vi "Config.vi"(8 "error in (no error)":errorcluster, 10 "Setting":variant, 11 "Lambda Gen LAN in":refnum<class "Lambda Gen LAN.lvclass">) -> (0 "error out":errorcluster, 3 "Lambda Gen LAN out":refnum<class "Lambda Gen LAN.lvclass">)   [LabVIEW 2025, in "Power Supply.lvlib" / "Lambda Gen LAN.lvclass"]
uses:
  Lambda Gen LAN.lvclass
  C:/Users/Public/Documents/Sandia National Labs/TSS Plugin/CEF.lvlibp/Node/CEF_Node.lvclass
  C:/Users/Public/Documents/Sandia National Labs/TSS Plugin/Abstract Engine.lvlibp/Abstract Instrument/Abstract Instrument.lvclass
  PS Channel/Power Supply Channel.lvclass
  Users/Public/Documents/Sandia National Labs/TSS Plugin/Abstract Engine.lvlibp/Abstract Instrument/Channel.ctl
  Lambda Gen LAN.lvclass/Lambda Gen LAN.ctl
  PS Channel configuration/Power Supply Channel configuration.lvclass
  C:/Users/Public/Documents/Sandia National Labs/TSS Plugin/Abstract Engine.lvlibp/Channel configuration/Channel configuration.lvclass
  PS Channel configuration/Power Supply Channel configuration.lvclass/Power Supply Channel configuration.ctl
  PS Channel configuration/Read PS Channel.vi
  Users/Public/Documents/Sandia National Labs/TSS Plugin/CEF.lvlibp/Node/ReadChildren.vi
  Users/Public/Documents/Sandia National Labs/TSS Plugin/Abstract Engine.lvlibp/Channel configuration/Read Channel Setting.vi
  Users/Public/Documents/Sandia National Labs/TSS Plugin/CEF.lvlibp/Node/CEF_Node.lvclass
  Users/Public/Documents/Sandia National Labs/TSS Plugin/CEF.lvlibp/serializable configuration/CEF_serializable configuration.lvclass
  <instrlib>/TDK-Lambda GEN LAN Series/TDK-Lambda GEN LAN Series.lvlib
  Users/Public/Documents/Sandia National Labs/TSS Plugin/Abstract Engine.lvlibp/Abstract Instrument/Abstract Instrument.lvclass
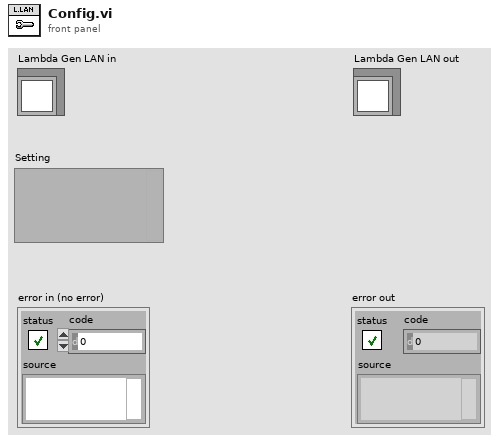
[diagram p1: front panel]
types:
  T1 = typedef "Abstract Engine.lvlibp/Abstract Instrument.lvclass/Channel.ctl" = cluster{"Alias":string, "DataType":enum16{"Anaolg Input", "Waveform"}, "Unit":enum16{"---", "V", "A", "Ohm", "Hz", "uF", "degC", "deg"}, "Upper limit":dbl, "Lower limit":dbl, "Measurement":variant}
  T2 = typedef "Abstract Engine.lvlibp/Channel configuration.lvclass/Default Channel.ctl" = cluster{"Address":string, "SW Alias":string, "Enabled":bool, "Type":string, "Description":string}
  T3 = typedef "Power Supply.lvlib/Power Supply Channel configuration.lvclass/PS Channel Setting.ctl" = cluster{"Driver":string, "Pin":string, "Test Voltage":string, "Voltage Low":dbl, "Voltage Norminal":dbl, "Voltage High":dbl, "PreTest Voltage":dbl, "PreTest Current":dbl, "Current Limit":dbl}
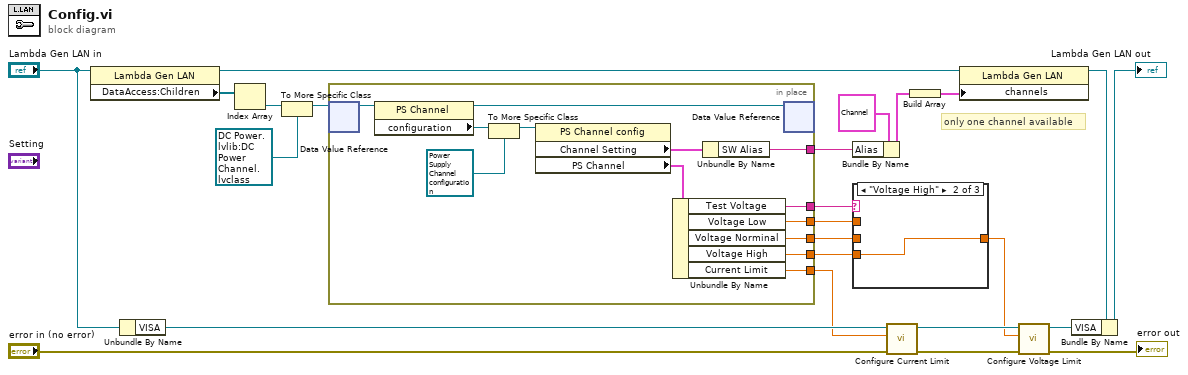
[diagram p0: block diagram]
diagram:
  # "only one channel available"
  n1 = property class="Lambda Gen LAN"(reference="Lambda Gen LAN in") -> (reference out=w18:refnum<class "Lambda Gen LAN.lvclass">, "DataAccess:Children"=w17:refnum<data-value>[])  [unwired: 1 in, 1 out]
  n2 = Unbundle By Name("Lambda Gen LAN in") -> ("VISA"=w23:refnum<visa-resource-name>)
  n3 = Index Array(array=w17) -> (element=w16:refnum<data-value>)  [unwired: 1 in]
  n4 = To More Specific Class(target class=refnum<data-value> refnum ("data value reference"), reference=w16) -> (specific class reference=w15:refnum<data-value>)  [unwired: 1 in, 1 out]
  n5 = in-place {
    in-place-border: [w29] -> w10
    in-place-border: [w30] -> w8
    in-place-border: [w28] -> w7
    in-place-border: [w27] -> w6
    in-place-border: [w26] -> w4
    in-place-border: [w25] -> w3
    # "Initialize the front panel controls when loaded"
    n6 = in-place-dvr #1(w15) -> (w37:refnum<class "Power Supply Channel.lvclass">)  [unwired: 1 out]
    n7 = property class="PS Channel"(reference=w37) -> (reference out=w36:refnum<class "Power Supply Channel.lvclass">, "configuration"=w35:refnum<class "CEF_serializable configuration.lvclass">)  [unwired: 1 in, 1 out]
    n8 = To More Specific Class(target class=refnum<class "Power Supply Channel configuration.lvclass"> refnum ("DC Power.lvlib:DCPower Channel configuration.lvclass"), reference=w35) -> (specific class reference=w34:refnum<class "Power Supply Channel configuration.lvclass">)  [unwired: 1 in, 1 out]
    n9 = property class="PS Channel config"(reference=w34) -> ("Channel Setting"=w31:T2, "PS Channel"=w32:T3)  [unwired: 1 in, 2 out]
    n10 = Unbundle By Name(w32) -> ("Test Voltage"=w28:string, "Voltage Low"=w26:dbl, "Voltage Norminal"=w27:dbl, "Voltage High"=w25:dbl, "Current Limit"=w29:dbl)
    n11 = Unbundle By Name(w31) -> ("SW Alias"=w30:string)
    n12 = in-place-dvr #1(w36) -> ()  [unwired: 2 out]
  }
  n13 = Bundle By Name(cluster=T1 {"Alias"="ch0", "DataType"=enum."Anaolg Input", "Unit"=enum."V", "Upper limit"=10.0, "Lower limit"=-10.0, "Measurement"=variant} ("Channel"), "Alias"=w8) -> (w9:T1)
  n14 = case shown="\"Voltage High\"" w7 {
    tunnel: w4 -> [_ _ w40]
    tunnel: w6 -> [w38 _ _]
    tunnel: w3 -> [_ w39 _]
    tunnel: [w38 w39 w40] -> w5
    frame "Voltage Norminal", Default {
    }
    frame "Voltage High" {
    }
    frame "Voltage Low" {
    }
  }
  n15 = call <instrlib>:"Configure Current Limit.vi"("error"="error in (no error)", "Current Limit"=w10, "VISA"=w23) -> ("error out"=w22:errorcluster, "VISA out"=w21:refnum<visa-resource-name>)  [unwired: 7 in]
  n16 = Build Array(w9) -> (w2:T1[])
  n17 = property class="Lambda Gen LAN"(reference=w18, "channels"=w2) -> (reference out=w11:refnum<class "Lambda Gen LAN.lvclass">)  [unwired: 1 in, 1 out]
  n18 = call <instrlib>:"Configure Voltage Limit.vi"("error"=w22, "Voltage Limit"=w5, "VISA"=w21) -> ("error out"=→"error out":errorcluster, "VISA out"=w20:refnum<visa-resource-name>)  [unwired: 7 in]
  n19 = Bundle By Name(cluster=w11, "VISA"=w20) -> (→"Lambda Gen LAN out":refnum<class "Lambda Gen LAN.lvclass">)
